vi "BCD_performance test.vi"() -> ()   [LabVIEW 2020]
uses:
  _Projects/1553 fabio/BCI-1553B/Source/Engine/BCI-1553B Engine.lvlib
panel:
  in  "Numeric 2":i32
  in  "Numeric":i32
  out "y 2":u32
  out "y":u32
  out "sum":u32
  out "decimal":dbl format="%.2f"
  out "raw bin":u16 format="%016b"
  in  "bcd":u16
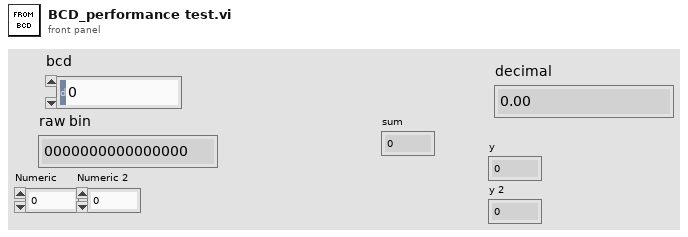
[diagram p1: front panel]
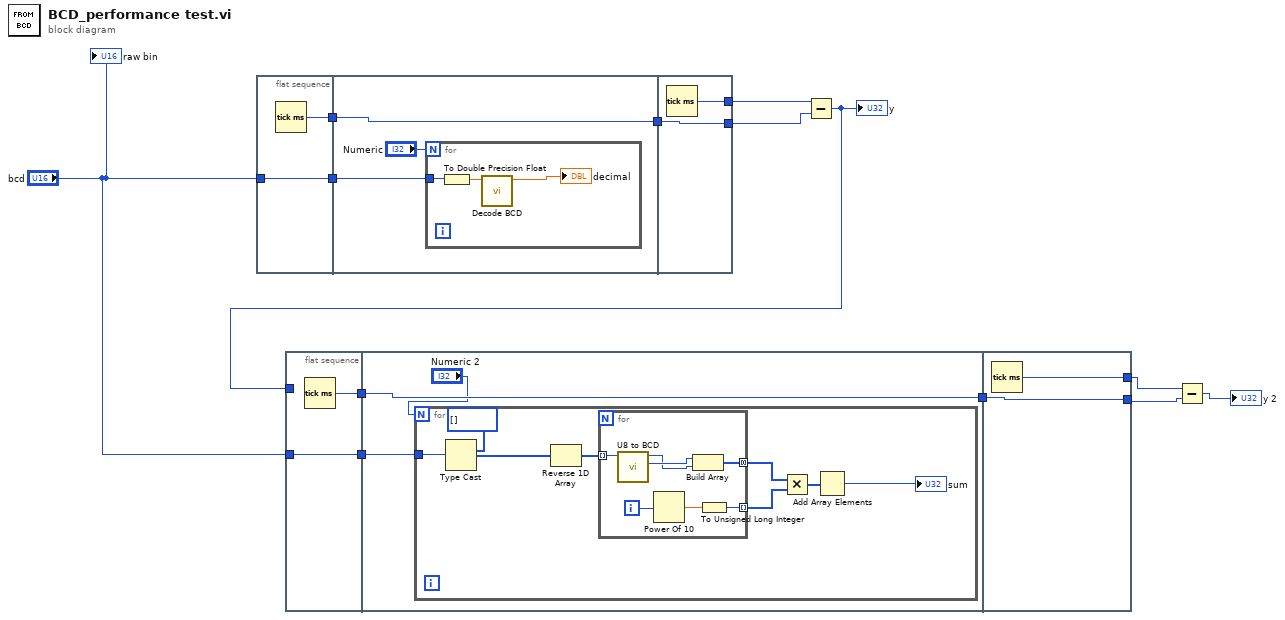
[diagram p0: block diagram]
diagram:
  n1 = flat-sequence {
    tunnel: "bcd" -> [w15]
    tunnel: [w15] -> w13
    tunnel: [w14] -> w12
    tunnel: w13 -> [w18]
    tunnel: w12 -> [w17]
    tunnel: [w17] -> w11
    tunnel: [w23] -> w10
    tunnel: [w22] -> w9
    tunnel: w11 -> [w22]
    frame #0 {
      n2 = Tick Count (ms)() -> (millisecond timer value=w14:u32)
    }
    frame #1 {
      n3 = for {
        N: "Numeric" -> [_]
        tunnel: w18 -> [w19]
        n4 = To Double Precision Float(number=w19) -> (double precision float=w21:dbl)
        n5 = call "Decode BCD.vi"("Data Raw"=w21) -> ("BCD Data"=→"decimal":dbl)  [unwired: 10 in]
      }
    }
    frame #2 {
      n6 = Tick Count (ms)() -> (millisecond timer value=w23:u32)
    }
  }
  n7 = flat-sequence {
    tunnel: "bcd" -> [w25]
    tunnel: [w25] -> w8
    tunnel: [w24] -> w7
    tunnel: w4 -> [_]
    tunnel: w8 -> [w28]
    tunnel: w7 -> [w27]
    tunnel: [w27] -> w6
    tunnel: [w45] -> w3
    tunnel: [w44] -> w2
    tunnel: w6 -> [w44]
    frame #0 {
      n8 = Tick Count (ms)() -> (millisecond timer value=w24:u32)
    }
    frame #1 {
      n9 = for {
        N: "Numeric 2" -> [_]
        tunnel: w28 -> [w29]
        n10 = Type Cast(type=u8[] [], x=w29) -> (*(type *) &x=w31:u8[])
        n11 = Reverse 1D Array(array=w31) -> (reversed array=w32:u8[])
        n12 = for {
          tunnel: w32 -> [w43] mode=indexing
          tunnel: [w37] -> w34 mode=indexing
          tunnel: [w38] -> w33 mode=concatenating
          i -> [w42]
          n13 = call "U8 to BCD.vi"("decimal in"=w43) -> ("low nibble"=w40:u8, "hi nibble"=w39:u8)  [unwired: 9 in]
          n14 = Power Of 10(x=w42) -> (10^x=w41:dbl)
          n15 = Build Array(w40, w39) -> (w38:u8[])
          n16 = To Unsigned Long Integer(number=w41) -> (unsigned 32bit integer=w37:u32)
        }
        n17 = Multiply(x=w33, y=w34) -> (x*y=w35:u32[])
        n18 = Add Array Elements(numeric array=w35) -> (sum=→"sum":u32)
      }
    }
    frame #2 {
      n19 = Tick Count (ms)() -> (millisecond timer value=w45:u32)
    }
  }
  n20 = Subtract(x=w10, y=w9) -> (x-y=w4:u32)
  "y" <- w4
  n21 = Subtract(x=w3, y=w2) -> (x-y=→"y 2":u32)
  "raw bin" <- "bcd"
